vi "NActiveBitsCounter.vi"(1 "Input Number":i32) -> (0 "N High Bits":i32)   [LabVIEW 2009]
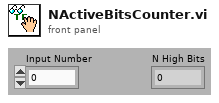
[diagram p1: front panel]
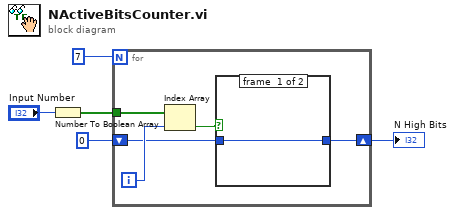
[diagram p0: block diagram]
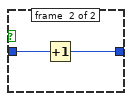
[diagram p2: hidden frame]
diagram:
  n1 = Number To Boolean Array(number="Input Number") -> (Boolean array=w5:bool[])
  n2 = for {
    N: 7 -> [_]
    tunnel: w5 -> [w10]
    shift-right: [w7] -> w4
    shift-left: u8 0 -> [w6]
    i -> [w8]
    n3 = Index Array(array=w10, index=w8) -> (element=w9:bool)
    n4 = case shown="True" w9 {
      tunnel: [w11 w13] -> w7
      tunnel: w6 -> [w11 w12]
      frame #0 {
      }
      frame #1 {
        n5 = Increment(x=w12) -> (x+1=w13:u8)
      }
    }
  }
  "N High Bits" <- w4
